vi "Start Stop Profile.vi"(0 "reference in":refnum<class "DCIR.lvclass">, 5 "Start Stop Profile":bool, 7 "Profile Complete Event":refnum<user-event>, 11 "Error In":errorcluster) -> (4 "reference out":refnum<class "DCIR.lvclass">, 15 "Error Out":errorcluster)   [LabVIEW 2023, in "DCIR.lvclass"]
uses:
  DCIR.lvclass
  DCIR.lvclass/DCIR.ctl
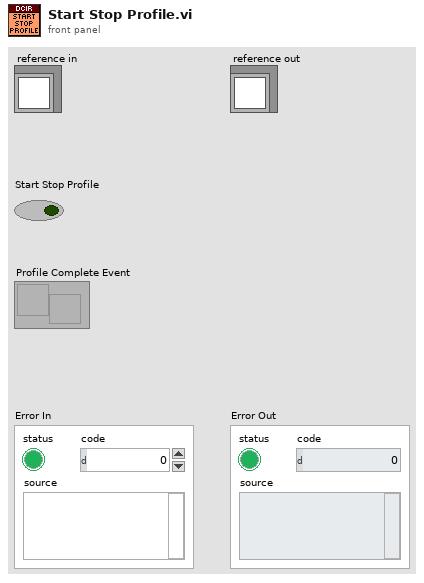
[diagram p1: front panel]
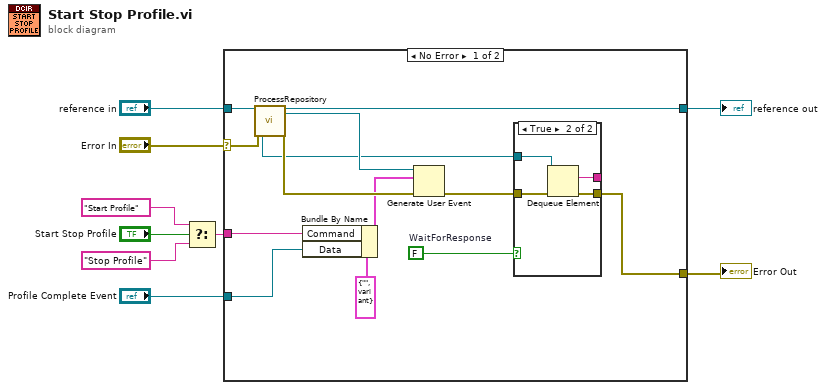
[diagram p0: block diagram]
diagram:
  n1 = Select(t="Start Profile" ("Command"), s="Start Stop Profile", f="Stop Profile" ("Command")) -> (s? t:f=w4:string)
  n2 = case shown="No Error" "Error In" {
    selector: "Error In" -> [w22 w29]
    tunnel: [w15 w29] -> w8
    tunnel: [w20 w28] -> w6
    tunnel: "reference in" -> [w21 w28]
    tunnel: w4 -> [w11 _]
    tunnel: "Profile Complete Event" -> [w10 _]
    frame No Error {
      w18 = FALSE  # WaitForResponse
      n3 = call "ProcessRepository.vi"("reference in"=w21, "Error In"=w22) -> ("QueueFromProcess"=w12:refnum<queue>, "reference out"=w20:refnum<class "DCIR.lvclass">, "EventsToProcess"=w19:refnum<user-event>, "Error Out"=w16:errorcluster)  [unwired: 10 in, 4 out]
      n4 = Bundle By Name(cluster=cluster{"Command":string, "Data":variant} {"Command"="", "Data"=variant} ("MessageToProcess"), "Command"=w11, "Data"=w10) -> (w13:cluster{"Command":string, "Data":variant})
      n5 = Generate User Event(user event=w19, event data cluster=w13, error in=w16) -> (error out=w17:errorcluster)  [unwired: 1 in, 1 out]
      n6 = case shown="True" w18 {
        tunnel: w17 -> [w23 w27]
        tunnel: [_ w26] -> _
        tunnel: [w23 w25] -> w15
        tunnel: w12 -> [_ w24]
        frame False {
        }
        frame True {
          n7 = Dequeue Element(queue=w24, error in (no error)=w27) -> (element=w26:string, error out=w25:errorcluster)  [unwired: 1 in, 2 out]
        }
      }
    }
    frame Error {
    }
  }
  "Error Out" <- w8
  "reference out" <- w6
